vi "Write to XML.vi"(8 "error in":errorcluster, 11 "Flattening in":refnum<class "Flattening.lvclass">) -> (0 "error out":errorcluster, 3 "Flattening out":refnum<class "Flattening.lvclass">)   [LabVIEW 2019, in "Flattening.lvclass"]
uses:
  Flattening.lvclass
  Flattening.lvclass/Flattening.ctl
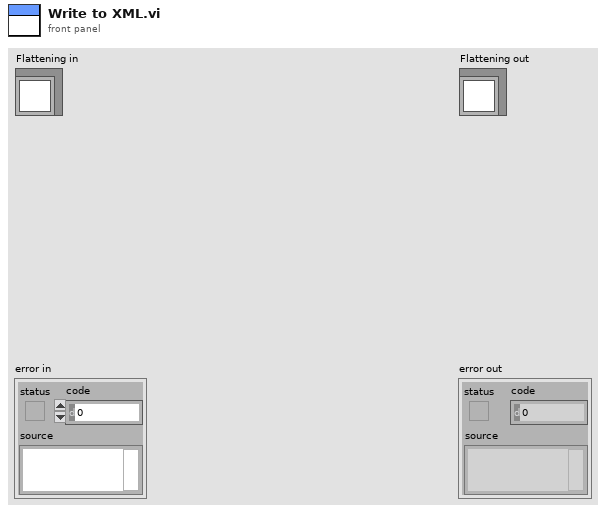
[diagram p1: front panel]
types:
  T1 = enum16{"open", "replace", "create", "open or create", "replace or create", "replace or create with confirmation"}
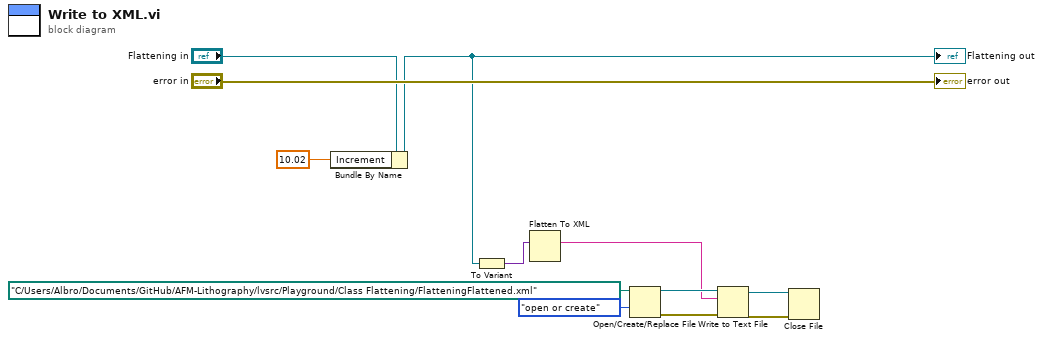
[diagram p0: block diagram]
diagram:
  n1 = Bundle By Name(cluster="Flattening in", "Increment"=10.02 ("DataValueHere")) -> (w2:refnum<class "Flattening.lvclass">)
  "Flattening out" <- w2
  n2 = To Variant(anything=w2) -> (Variant=w1:variant)
  n3 = Flatten To XML(anything=w1) -> (xml string=w4:string)
  n4 = Open/Create/Replace File(file path (use dialog)=path "C:/Users/Albro/Documents/GitHub/AFM-Lithography/lvsrc/Playground/Class Flattening/FlatteningFlattened.xml", operation (0:open)=T1."open or create") -> (refnum out=w9:refnum<file>, error out=w8:errorcluster)  [unwired: 4 in, 1 out]
  n5 = Write to Text File(file (use dialog)=w9, text=w4, error in=w8) -> (refnum out=w7:refnum<file>, error out=w6:errorcluster)  [unwired: 1 in, 1 out]
  n6 = Close File(refnum=w7, error in=w6) -> ()  [unwired: 2 out]
  "error out" <- "error in"
